vi "testVisa.vi"() -> ()   [LabVIEW 2026]
uses:
  <userlib>/Sensor.ctl
  <vilib>/Instr/_visa.llb/VISA Configure Serial Port (Instr).vi
panel:
  out "Waveform Graph":waveform(dbl)(graph)
  in  "stop":bool
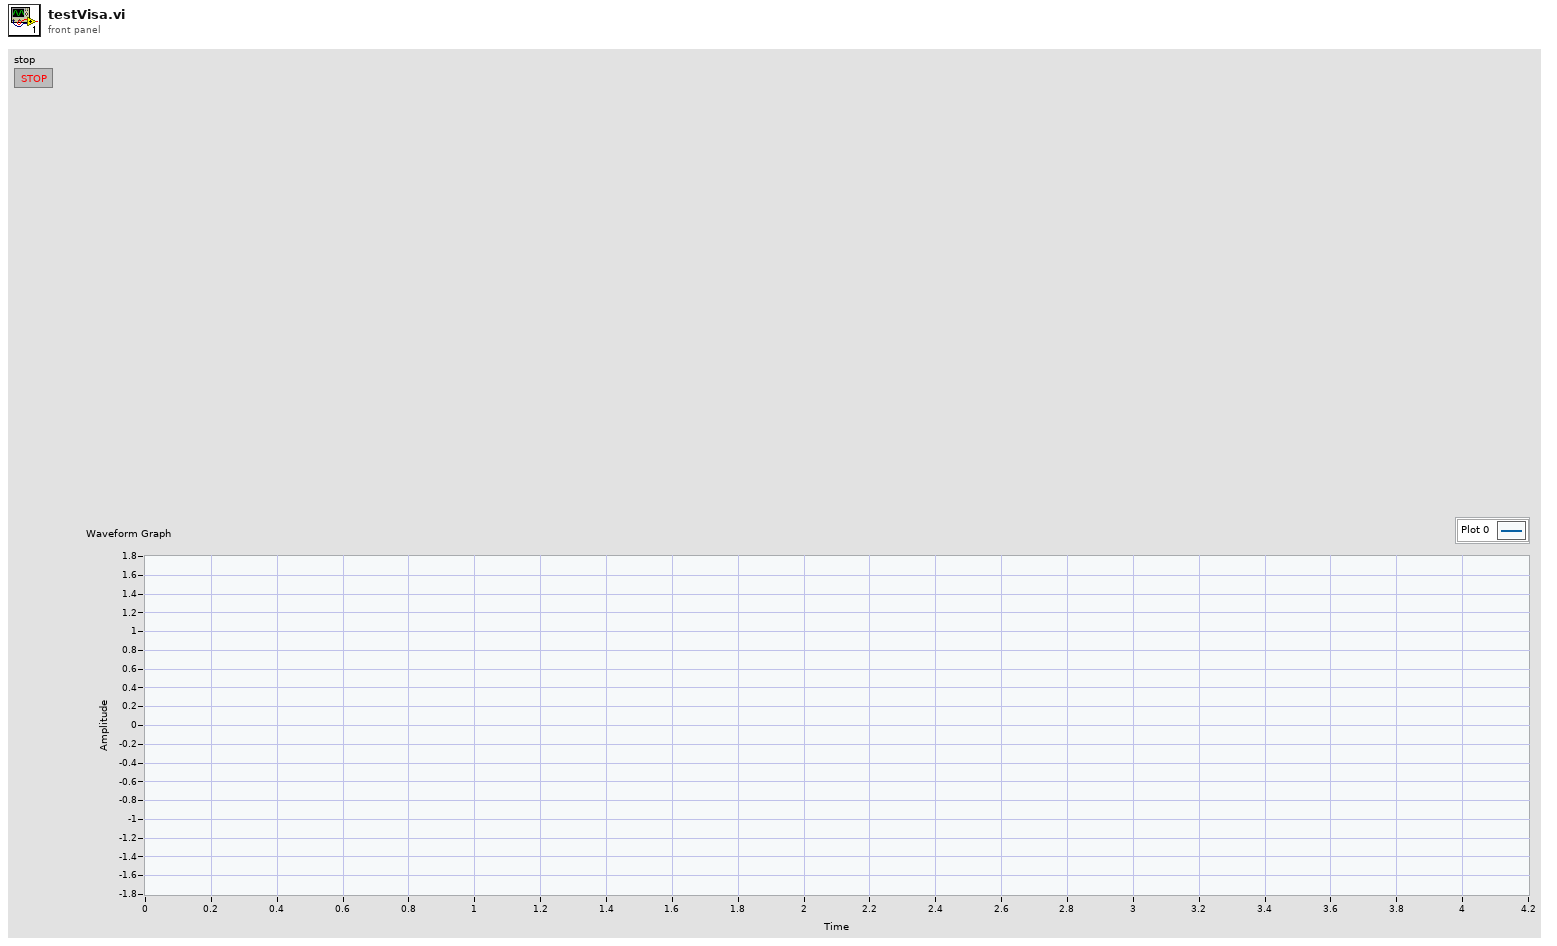
[diagram p1: front panel]
types:
  T1 = typedef "Sensor.ctl" = enum16{"EMG", "ECG", "EEG", "EDA", "ACC", "LUX"}
  T2 = cluster{"Sensor 1":T1, "Sensor 2":T1, "Sensor 3":T1, "Sensor 4":T1, "Sensor 5":T1, "Sensor 6":T1}
  T3 = cluster{"Result":dbl, "Result":dbl, "Result":dbl, "Result":dbl, "Result":dbl, "Result":dbl}
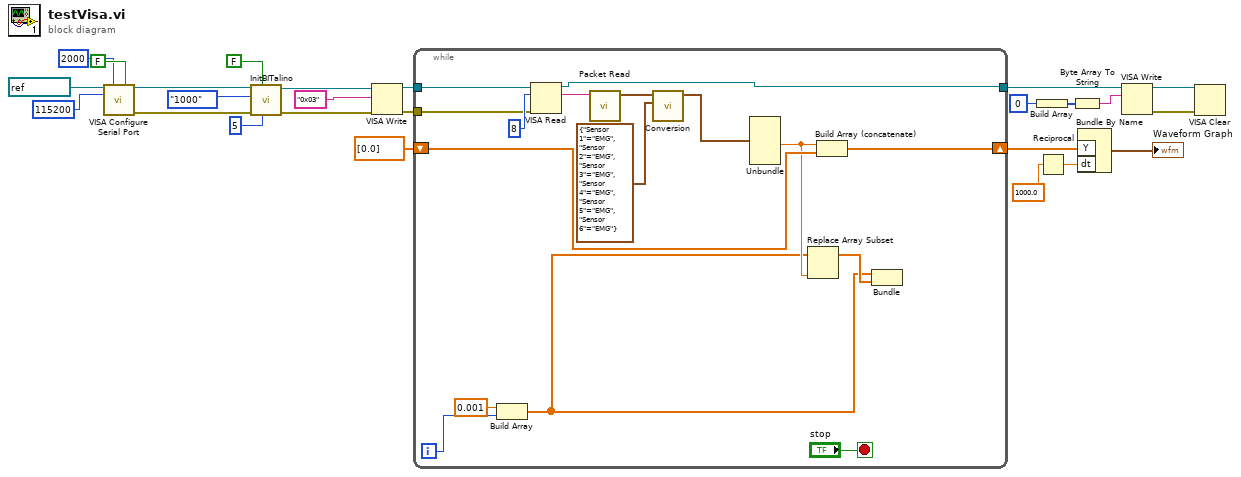
[diagram p0: block diagram]
diagram:
  n1 = call-poly "VISA Configure Serial Port"("VISA resource name"=refnum<visa-resource-name> "COM3", "timeout (10sec)"=u32 2000, "Enable Termination\nChar (T)"=FALSE ("Enable Termination\nChar (T)"), "baud rate (9600)"=u32 115200) -> ("VISA resource name out"=w22:refnum<visa-resource-name>, "error out"=w21:errorcluster)  [unwired: 10 in]
  n2 = call "InitBITalino.vi"("Battery \nThreshold (%)"=u8 5 ("Battery \nThreshold (%)"), "MODE"=FALSE, "error in (no error)"=w21, "Sample Rate"=enum16{"1", "10", "100", "1000"}."1000", "BITalino"=w22) -> ("error out"=w11:errorcluster, "VISA out"=w9:refnum<visa-resource-name>)  [unwired: 4 in, 1 out]
  n3 = VISA Write(VISA resource name=w9, write buffer="0x03", error in (no error)=w11) -> (VISA resource name out=w7:refnum<visa-resource-name>, error out=w8:errorcluster)  [unwired: 1 out]
  n4 = while {
    tunnel: [w37] -> w20
    tunnel: w8 -> [w35]
    tunnel: w7 -> [w34]
    shift-right: [w32] -> w5
    shift-left: dbl[] [0.0] -> [w31]
    i -> [w30]
    stop <- "stop" stop-if-true
    n5 = Build Array(0.001 ("element"), w30) -> (w26:dbl[])
    n6 = VISA Read(VISA resource name=w34, byte count=u32 8, error in (no error)=w35) -> (VISA resource name out=w37:refnum<visa-resource-name>, read buffer=w40:string)  [unwired: 2 out]
    n7 = call "Packet Read.vi"("Packets"=w40) -> ("Analog Channels"=w39:cluster{u16, u16, u16, u16, u16, u16})  [unwired: 7 in, 3 out]
    n8 = call "Conversion.vi"("Sensor Type"=T2 {"Sensor 1"=enum."EMG", "Sensor 2"=enum."EMG", "Sensor 3"=enum."EMG", "Sensor 4"=enum."EMG", "Sensor 5"=enum."EMG", "Sensor 6"=enum."EMG"}, "Analog Channels"=w39) -> ("Converted Values"=w33:T3)  [unwired: 8 in, 1 out]
    n9 = Unbundle(w33) -> ("Result"=w28:dbl)  [unwired: 5 out]
    n10 = Replace Array Subset(array=w26, new element=w28) -> (w27:dbl[])  [unwired: 1 in]
    n11 = Build Array (concatenate)(w28, w31) -> (w32:dbl[])
    n12 = Bundle(w26, w27) -> ()  [unwired: 1 in, 1 out]
  }
  n13 = Build Array(u8 0) -> (w16:u8[])
  n14 = Reciprocal(x=1000.0) -> (1/x=w4:dbl)
  n15 = Byte Array To String(unsigned byte array=w16) -> (string=w15:string)
  n16 = Bundle By Name("Y"=w5, "dt"=w4) -> (→"Waveform Graph":waveform(dbl))  [unwired: 1 in]
  n17 = VISA Write(VISA resource name=w20, write buffer=w15) -> (VISA resource name out=w19:refnum<visa-resource-name>, error out=w18:errorcluster)  [unwired: 1 in, 1 out]
  n18 = VISA Clear(VISA resource name=w19, error in (no error)=w18) -> ()  [unwired: 2 out]
